vi "Publish AI.vi"(8 "error in":errorcluster, 10 "AI Data":dbl[](array[numeric]), 11 "BNT_ULx-MCSV in":refnum<class "BNT_ULx-MCSV.lvclass">) -> (0 "error out":errorcluster, 3 "BNT_ULx-MCSV out":refnum<class "BNT_ULx-MCSV.lvclass">)   [LabVIEW 2021, in "BNT_ULx.lvlib" / "BNT_ULx-MCSV.lvclass"]
doc: "Publish analog input values if greater than uncertainty."
uses:
  BNT_ULx-MCSV.lvclass
  BNT_ULx-MCSV.lvclass/BNT_ULx-MCSV.ctl
  CSPP_Core/Classes/CSPP_ProcessVariables/PVConnection/PVConnection.lvclass/PVConnection.ctl
  CSPP_Core/Classes/CSPP_ProcessVariables/ProcessVariable/PV.lvclass/PV.ctl
  CSPP_Core/Classes/CSPP_ProcessVariables/ProcessVariable/Write Data.vi
  CSPP_Core/Classes/CSPP_ProcessVariables/ProcessVariable/Write Error.vi
  CSPP_Core/Classes/CSPP_ProcessVariables/ProcessVariable/Write Quality.vi
  CSPP_Core/Classes/CSPP_ProcessVariables/ProcessVariable/Write status.vi
  CSPP_Core/Classes/CSPP_ProcessVariables/ProcessVariable/Write Timestamp.vi
  CSPP_Core/Classes/CSPP_ProcessVariables/ProcessVariable/PV.lvclass
  CSPP_Core/Classes/CSPP_ProcessVariables/PVConnection/PVConnection.lvclass
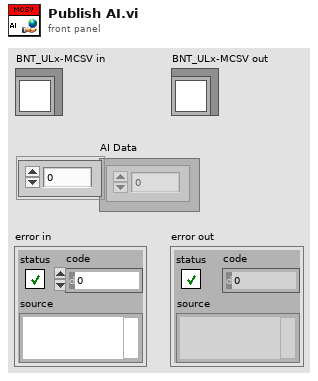
[diagram p1: front panel]
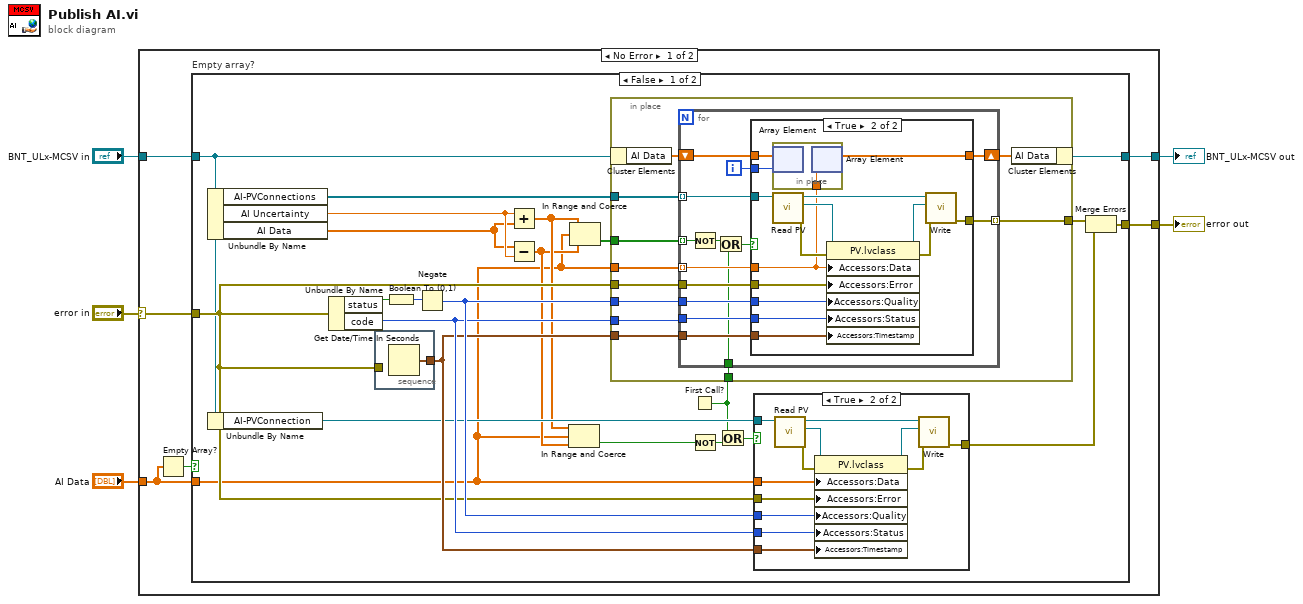
[diagram p0: block diagram]
diagram:
  n1 = case shown="No Error" "error in" {
    selector: "error in" -> [w11 w95]
    tunnel: [w10 w95] -> w4
    tunnel: [w8 w94] -> w2
    tunnel: "BNT_ULx-MCSV in" -> [w9 w94]
    tunnel: "AI Data" -> [w6 _]
    frame No Error {
      n2 = Empty Array?(array=w6) -> (empty?=w7:bool)
      n3 = case "Empty array?" shown="False" w7 {
        tunnel: w11 -> [w27 w92]
        tunnel: [w25 w92] -> w10
        tunnel: w6 -> [w14 _]
        tunnel: w9 -> [w18 w93]
        tunnel: [w17 w93] -> w8
        frame False {
          n4 = Unbundle By Name(w18) -> ("AI-PVConnections"=w26:refnum<class "PVConnection.lvclass">[], "AI Uncertainty"=w23:dbl, "AI Data"=w21:dbl[])
          n5 = Unbundle By Name(w18) -> ("AI-PVConnection"=w24:refnum<class "PVConnection.lvclass">)
          n6 = Unbundle By Name(w27) -> ("status"=w33:bool, "code"=w30:i32)
          n7 = stacked-sequence {
            tunnel: [w78] -> w29
            tunnel: w27 -> [_]
            frame #0 {
              n8 = Get Date/Time In Seconds() -> (seconds since 1Jan1904=w78:timestamp)
            }
          }
          n9 = Boolean To (0,1)(Boolean=w33) -> (0, 1=w32:i16)
          n10 = Negate(x=w32) -> (-x=w31:i16)
          n11 = Add(x=w23, y=w21) -> (x+y=w20:dbl[])
          n12 = Subtract(x=w21, y=w23) -> (x-y=w19:dbl[])
          n13 = In Range and Coerce(upper limit=w20, x=w14, lower limit=w19) -> (In Range?=w16:bool)  [unwired: 1 out]
          n14 = In Range and Coerce(upper limit=w20, x=w14, lower limit=w19) -> (In Range?=w22:bool[])  [unwired: 1 out]
          n15 = First Call?() -> (First Call?: T/F=w13:bool)
          n16 = in-place {
            in-place-border: [w45] -> w34
            in-place-border: w31 -> [w44]
            in-place-border: w30 -> [w43]
            in-place-border: w29 -> [w42]
            in-place-border: w27 -> [w41]
            in-place-border: w26 -> [w40]
            in-place-border: w14 -> [w39]
            in-place-border: w22 -> [w38]
            in-place-border: w13 -> [w35]
            n17 = in-place-cluster #1(w18) -> ("AI Data"=w37:dbl[])
            n18 = for {
              tunnel: w40 -> [w53] mode=indexing
              tunnel: w39 -> [w59] mode=indexing
              tunnel: w41 -> [w58]
              tunnel: [w57] -> w45 mode=indexing
              tunnel: w44 -> [w56]
              tunnel: w43 -> [w55]
              tunnel: w42 -> [w54]
              tunnel: w38 -> [w52] mode=indexing
              shift-right: [w49] -> w36
              shift-left: w37 -> [w50]
              tunnel: w35 -> [w47]
              i -> [w51]
              n19 = Not(x=w52) -> (.not. x?=w46:bool)
              n20 = Or(x=w46, y=w47) -> (x .or. y?=w48:bool)
              n21 = case shown="True" w48 {
                tunnel: w59 -> [_ w63]
                tunnel: w58 -> [w61 w76]
                tunnel: [w61 w73] -> w57
                tunnel: w56 -> [_ w72]
                tunnel: w55 -> [_ w71]
                tunnel: w54 -> [_ w70]
                tunnel: w53 -> [_ w69]
                tunnel: w51 -> [_ w65]
                tunnel: w50 -> [w60 w64]
                tunnel: [w60 w62] -> w49
                frame False {
                }
                frame True {
                  n22 = in-place {
                    in-place-border: w63 -> [w77]
                    n23 = in-place-array #2(w64, w65) -> ()  [unwired: 1 out]
                    n24 = in-place-array #2(w77) -> (w62:dbl[])  [unwired: 1 out]
                  }
                  n25 = call "Read PV.vi"("PVConnection in"=w69) -> ("error out"=w66:errorcluster, "PV"=w67:refnum<class "PV.lvclass">, "PVConnection out"=w68:refnum<class "PVConnection.lvclass">)  [unwired: 8 in]
                  n26 = property class="PV.lvclass"(reference=w67, error in=w66, "Accessors:Data"=w63, "Accessors:Error"=w76, "Accessors:Quality"=w72, "Accessors:Status"=w71, "Accessors:Timestamp"=w70) -> (reference out=w75:refnum<class "PV.lvclass">, error out=w74:errorcluster)
                  n27 = call "Write.vi"("error in (no error)"=w74, "PV"=w75, "PVConnection in"=w68) -> ("error out"=w73:errorcluster)  [unwired: 6 in, 2 out]
                }
              }
            }
            n28 = in-place-cluster #1("AI Data"=w36) -> (w17:refnum<class "BNT_ULx-MCSV.lvclass">)
          }
          n29 = Not(x=w16) -> (.not. x?=w12:bool)
          n30 = Or(x=w13, y=w12) -> (x .or. y?=w15:bool)
          n31 = case shown="True" w15 {
            tunnel: w31 -> [_ w86]
            tunnel: w30 -> [_ w85]
            tunnel: w29 -> [_ w84]
            tunnel: [w79 w83] -> w28
            tunnel: w27 -> [w79 w82]
            tunnel: w24 -> [_ w81]
            tunnel: w14 -> [_ w80]
            frame False {
            }
            frame True {
              n32 = call "Read PV.vi"("PVConnection in"=w81) -> ("error out"=w87:errorcluster, "PV"=w88:refnum<class "PV.lvclass">, "PVConnection out"=w89:refnum<class "PVConnection.lvclass">)  [unwired: 8 in]
              n33 = property class="PV.lvclass"(reference=w88, error in=w87, "Accessors:Data"=w80, "Accessors:Error"=w82, "Accessors:Quality"=w86, "Accessors:Status"=w85, "Accessors:Timestamp"=w84) -> (reference out=w91:refnum<class "PV.lvclass">, error out=w90:errorcluster)
              n34 = call "Write.vi"("error in (no error)"=w90, "PV"=w91, "PVConnection in"=w89) -> ("error out"=w83:errorcluster)  [unwired: 6 in, 2 out]
            }
          }
          n35 = Merge Errors(w34, w28) -> (w25:errorcluster)
        }
        frame True {
        }
      }
    }
    frame Error {
    }
  }
  "error out" <- w4
  "BNT_ULx-MCSV out" <- w2
